vi "XBee String to Queue.vi"(8 "error in (no error)":errorcluster, 10 "String Received":string, 11 "Queue cluster":T3) -> (0 "error out":errorcluster, 3 "Battery Volts":dbl)   [LabVIEW 2013]
doc: "This VI takes in the queue cluster and an XBee string, then writes that data to the correct queues.\n\nEric Schneider, April 2014"
uses:
  Data/TypeDefs/GPS-Compass Queue Cluster.ctl
  Data/TypeDefs/UTM Location.ctl
  Data/TypeDefs/WindData Queue Cluster.ctl
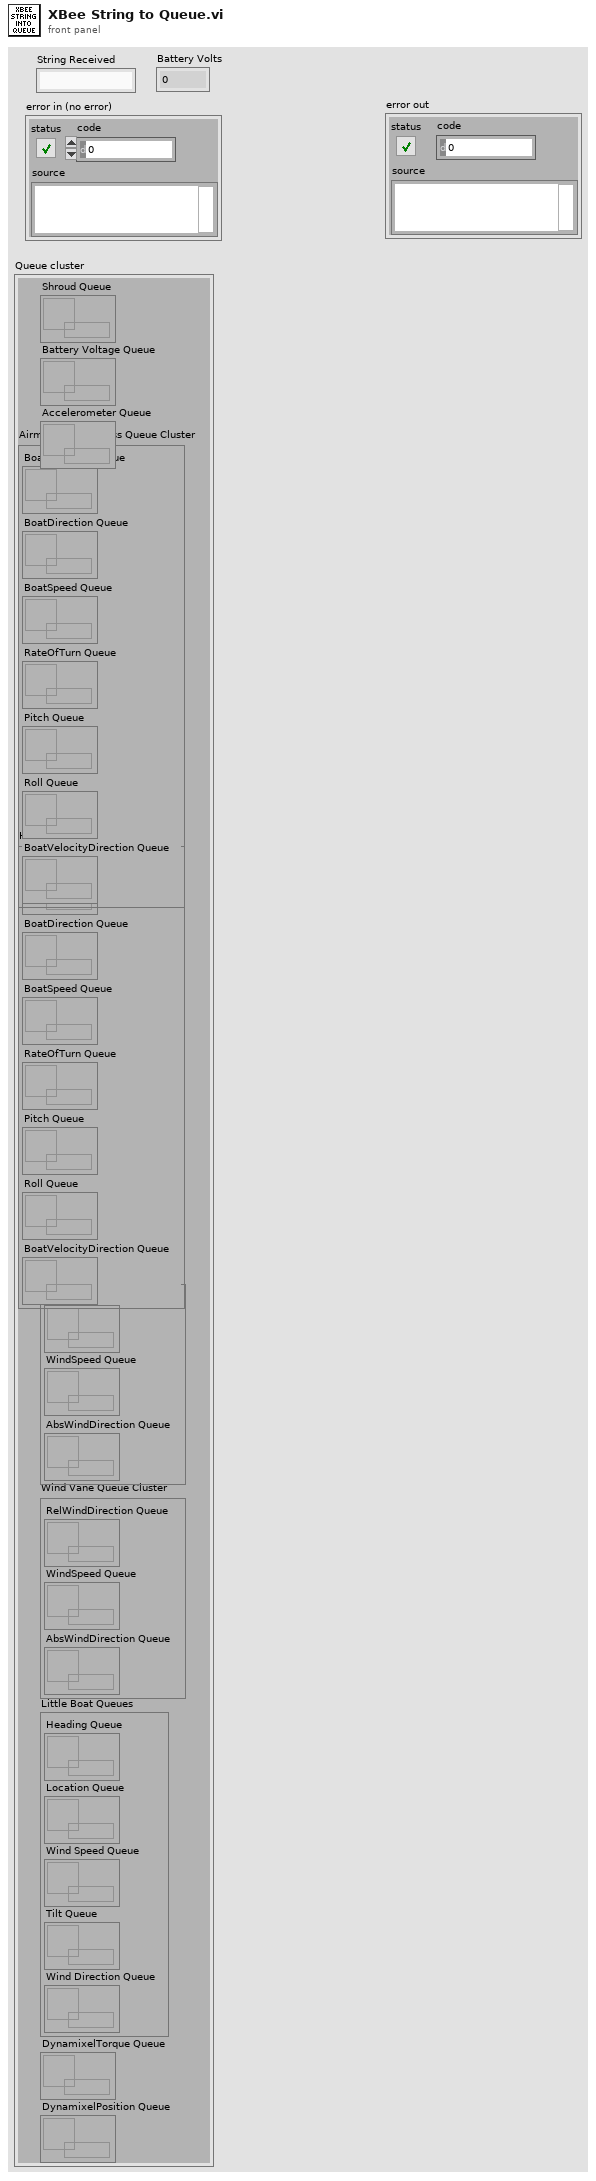
[diagram p1: front panel]
types:
  T1 = typedef "GPS-Compass Queue Cluster.ctl" = cluster{"BoatLocation Queue":refnum<queue>, "BoatDirection Queue":refnum<queue>, "BoatSpeed Queue":refnum<queue>, "RateOfTurn Queue":refnum<queue>, "Pitch Queue":refnum<queue>, "Roll Queue":refnum<queue>, "BoatVelocityDirection Queue ":refnum<queue>}
  T2 = typedef "WindData Queue Cluster.ctl" = cluster{"RelWindDirection Queue":refnum<queue>, "WindSpeed Queue":refnum<queue>, "AbsWindDirection Queue":refnum<queue>}
  T3 = cluster{"Shroud Queue":refnum<queue>, "Battery Voltage Queue":refnum<queue>, "Accelerometer Queue":refnum<queue>, "AirmarGPS-Compass Queue Cluster":T1, "Hemisphere Queue Cluster":T1, "Airmar Wind Queue Cluster":T2, "Wind Vane Queue Cluster":T2, "Little Boat Queues":cluster{"Heading Queue":refnum<queue>, "Location Queue":refnum<queue>, "Wind Speed Queue":refnum<queue>, "Tilt Queue":refnum<queue>, "Wind Direction Queue":refnum<queue>}, "DynamixelTorque Queue":refnum<queue>, "DynamixelPosition Queue":refnum<queue>}
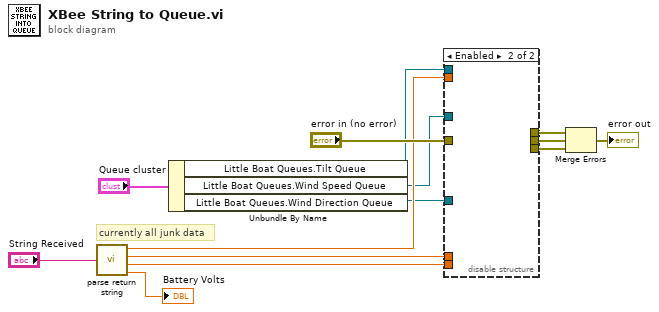
[diagram p0: block diagram]
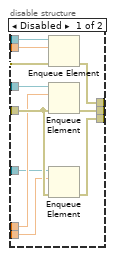
[diagram p2: hidden frame]
diagram:
  # "currently all junk data"
  n1 = call "parse return string.vi"("Return String"="String Received") -> ("Tilt"=w11:dbl, "Wind Speed"=w9:dbl, "Wind Direction"=w7:dbl, "Battery Volts"=→"Battery Volts":dbl)
  n2 = Unbundle By Name("Queue cluster") -> ("Little Boat Queues.Tilt Queue"=w12:refnum<queue>, "Little Boat Queues.Wind Speed Queue"=w10:refnum<queue>, "Little Boat Queues.Wind Direction Queue"=w8:refnum<queue>)
  n3 = disable-structure shown="Enabled" {
    disable-tunnel: "error in (no error)" -> [w24 _]
    disable-tunnel: w12 -> [w23 _]
    disable-tunnel: w11 -> [w22 _]
    disable-tunnel: w10 -> [w21 _]
    disable-tunnel: w9 -> [w20 _]
    disable-tunnel: w8 -> [w19 _]
    disable-tunnel: w7 -> [w18 _]
    disable-tunnel: [w17 _] -> w5
    disable-tunnel: [w16 _] -> w4
    disable-tunnel: [w15 _] -> w3
    frame Disabled {
      n4 = Enqueue Element(queue=w23, element=w22, error in (no error)=w24) -> (error out=w16:errorcluster)  [unwired: 1 in, 2 out]
      n5 = Enqueue Element(queue=w21, element=w20, error in (no error)=w24) -> (error out=w17:errorcluster)  [unwired: 1 in, 2 out]
      n6 = Enqueue Element(queue=w19, element=w18, error in (no error)=w24) -> (error out=w15:errorcluster)  [unwired: 1 in, 2 out]
    }
    frame Enabled {
    }
  }
  n7 = Merge Errors(w4, w5, w3) -> (→"error out":errorcluster)
